vi "ChannelType_Image.vi"(9 "error in":errorcluster, 11 "Image Reference":T2) -> (1 "error out":errorcluster, 2 "ChannelType":T1, 3 "Image Reference":T2)   [LabVIEW 2020, in "OpenLvVision_OpenCv.lvlib"]
uses:
  OpenLvVision_OpenCv.lvlib
  <vilib>/OpenLvVision/OpenLvVision_Image/Management/TypeDef/OLV Image.ctl
  <vilib>/OpenLvVision/OpenLvVision_Image/Management/TypeDef/OLV ImageType.ctl
  <vilib>/Utility/error.llb/Error Cluster From Error Code.vi
  <vilib>/ErrorRing/Error Ring.xnode
  <vilib>/OpenLvVision/OpenLvVision_Image/Management/OLV Management.lvlib
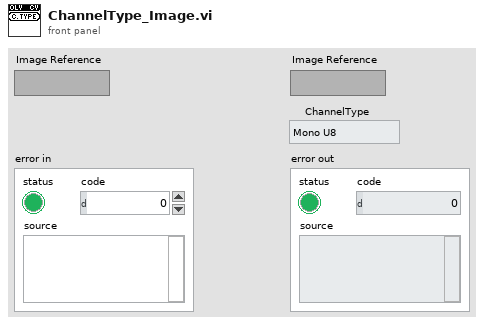
[diagram p1: front panel]
types:
  T1 = typedef "OLV OpenLvVision_Image.lvlib/OLV Management.lvlib/OLV ImageType.ctl" = enum16{"Mono U8", "Mono U16", "Mono I16", "Mono SGL", "Color U32", "Color U64", "Complex CSG"}
  T2 = typedef "OLV OpenLvVision_Image.lvlib/OLV Management.lvlib/OLV Image.ctl" = refnum<image>
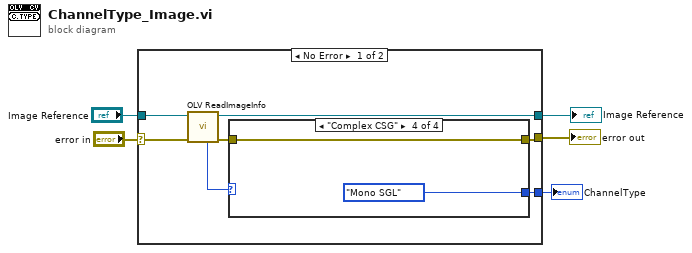
[diagram p0: block diagram]
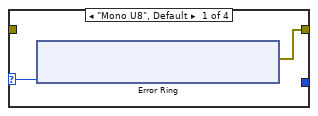
[diagram p2: hidden frame]
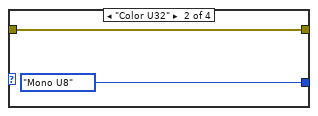
[diagram p3: hidden frame]
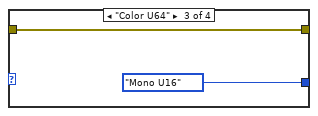
[diagram p4: hidden frame]
diagram:
  n1 = case shown="No Error" "error in" {
    selector: "error in" -> [w11 w28]
    tunnel: "Image Reference" -> [w12 w29]
    tunnel: [w10 w29] -> w3
    tunnel: [w6 w28] -> w2
    tunnel: [w8 _] -> w1
    frame No Error {
      n2 = call <vilib>:"OLV ReadImageInfo.vi"("error in"=w11, "Image Reference In"=w12) -> ("error out"=w7:errorcluster, "Image Reference Out"=w10:T2, "Image Type"=w9:T1)  [unwired: 4 in, 3 out]
      n3 = case shown="\"Complex CSG\"" w9 {
        selector: w9 -> [w13 _ _ _]
        tunnel: [_ OLV_ImageType."Mono U8" ("Image Type") OLV_ImageType."Mono U16" ("Image Type") OLV_ImageType."Mono SGL" ("Image Type")] -> w8
        tunnel: w7 -> [_ w22 w24 w27]
        tunnel: [w14 w22 w24 w27] -> w6
        frame "Mono U8", Default {
          n4 = xnode "Error Ring"("parameter 0"=w13) -> ("error out"=w14:errorcluster)
        }
        frame "Color U32" {
        }
        frame "Color U64" {
        }
        frame "Complex CSG" {
        }
      }
    }
    frame Error {
    }
  }
  "Image Reference" <- w3
  "error out" <- w2
  "ChannelType" <- w1
